vi "ReadSymbolCatalog.vi"(8 "error in (no error)":errorcluster, 11 "AdsNET in":refnum<class "AdsNET.lvclass">) -> (0 "error out":errorcluster, 3 "AdsNET out":refnum<class "AdsNET.lvclass">)   [LabVIEW 2016, in "TCatAdsNet.lvlib" / "AdsNET.lvclass"]
doc: "Reads symbol names and properties."
uses:
  AdsNET.lvclass
  AdsNET.lvclass/AdsNET.ctl
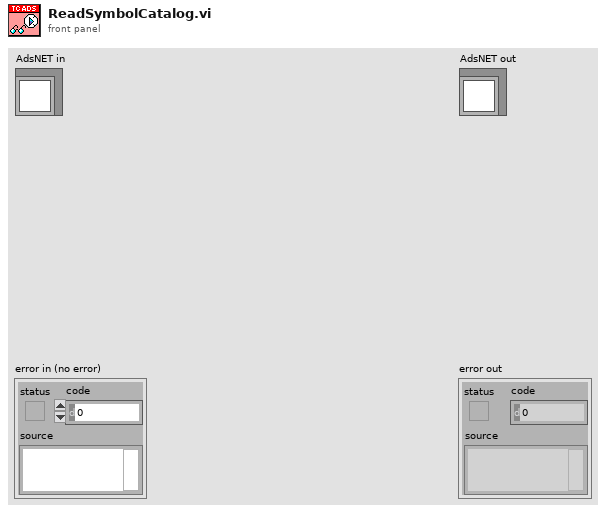
[diagram p1: front panel]
types:
  T1 = cluster{"Name":string, "IndexGroup":i64, "IndexOffset":i64, "Size":i32, "Type":string, "Datatype":i32, "Comment":string}
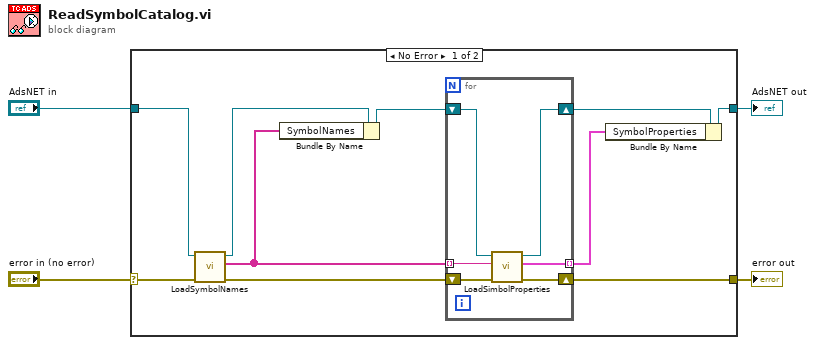
[diagram p0: block diagram]
diagram:
  n1 = case shown="No Error" "error in (no error)" {
    selector: "error in (no error)" -> [w12 w22]
    tunnel: [w8 w22] -> w3
    tunnel: [w6 w21] -> w1
    tunnel: "AdsNET in" -> [w14 w21]
    frame No Error {
      n2 = call "LoadSymbolNames.vi"("error in (no error)"=w12, "TCatAdsNet in"=w14) -> ("error out"=w9:errorcluster, "SymbolNameList"=w7:string[], "TCatAdsNet out"=w13:refnum<class "AdsNET.lvclass">)  [unwired: 7 in]
      n3 = Bundle By Name(cluster=w13, "SymbolNames"=w7) -> (w11:refnum<class "AdsNET.lvclass">)
      n4 = for {
        shift-right: [w19] -> w10
        shift-left: w11 -> [w20]
        shift-right: [w17] -> w8
        shift-left: w9 -> [w18]
        tunnel: w7 -> [w16] mode=indexing
        tunnel: [w15] -> w5 mode=indexing
        n5 = call "LoadSimbolProperties.vi"("error in (no error)"=w18, "name"=w16, "TCatAdsNet in"=w20) -> ("error out"=w17:errorcluster, "SymbolProperties"=w15:T1, "TCatAdsNet out"=w19:refnum<class "AdsNET.lvclass">)  [unwired: 5 in, 1 out]
      }
      n6 = Bundle By Name(cluster=w10, "SymbolProperties"=w5) -> (w6:refnum<class "AdsNET.lvclass">)
    }
    frame Error {
    }
  }
  "error out" <- w3
  "AdsNET out" <- w1
